vi "KGN Init.vi"(8 "Fehler (Eingang, kein Fehler)":errorcluster, 11 "VISA-Ressourcenname":refnum<visa-resource-name>) -> (0 "Fehler (Ausgang)":errorcluster, 2 "Device":string, 3 "VISA-Ressourcenname (Ausgang)":refnum<visa-resource-name>)   [LabVIEW 2020, in "Linearisierung v2.lvlib" / "Gasteiler.lvlib" / "HovaCAL_Interface.lvlib" / "KGN.lvlib"]
uses:
  KGN.lvlib
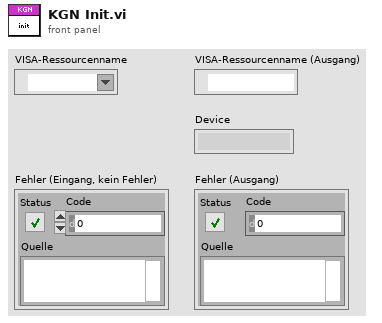
[diagram p1: front panel]
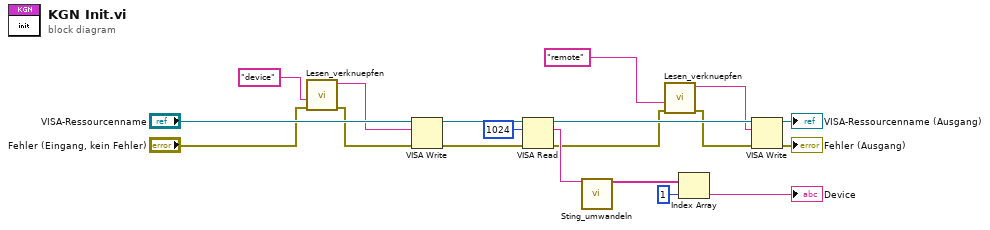
[diagram p0: block diagram]
diagram:
  n1 = call "Lesen_verknuepfen.vi"("error in (no error)"="Fehler (Eingang, kein Fehler)", "Order"="device" ("Schreibpuffer")) -> ("error out"=w10:errorcluster, "Verknüpfter String"=w4:string)  [unwired: 8 in]
  n2 = VISA Write(VISA resource name="VISA-Ressourcenname", write buffer=w4, error in (no error)=w10) -> (VISA resource name out=w19:refnum<visa-resource-name>, error out=w18:errorcluster)  [unwired: 1 out]
  n3 = VISA Read(VISA resource name=w19, byte count=u32 1024 ("Byte-Anzahl"), error in (no error)=w18) -> (VISA resource name out=w15:refnum<visa-resource-name>, read buffer=w14:string, error out=w8:errorcluster)  [unwired: 1 out]
  n4 = call "Sting_umwandeln.vi"("Lesepuffer"=w14) -> ("string array"=w2:string[])  [unwired: 8 in, 6 out]
  n5 = call "Lesen_verknuepfen.vi"("error in (no error)"=w8, "Order"="remote" ("Schreibpuffer")) -> ("error out"=w7:errorcluster, "Verknüpfter String"=w5:string)  [unwired: 8 in]
  n6 = Index Array(array=w2, index=1 ("Index")) -> (element=→"Device":string)
  n7 = VISA Write(VISA resource name=w15, write buffer=w5, error in (no error)=w7) -> (VISA resource name out=→"VISA-Ressourcenname (Ausgang)":refnum<visa-resource-name>, error out=→"Fehler (Ausgang)":errorcluster)  [unwired: 1 out]
